vi "Create Plot Object.vi"(6 "Control Ref Queue":T1, 7 "Actual Transform In":T2, 8 "error in (no error)":errorcluster, 9 "Multiplot Representation In":T4, 10 "3D Stem.lvclass in":refnum<class "3D Scatter.lvclass">, 11 "Plot Object In":refnum<vi>) -> (0 "error out":errorcluster, 1 "Multiplot Representation Out":T4, 2 "3D Stem.lvclass out":refnum<class "3D Scatter.lvclass">, 3 "Plot Object Out":refnum<vi>, 5 "Actual Transform Out":T2)   [LabVIEW 2020, in "3D Scatter.lvclass"]
uses:
  <vilib>/Math Plots/3D Math Plots/3D Scatter/3D Scatter/3D Scatter.lvclass
  <vilib>/Math Plots/3D Math Plots/3D Plot/3D Plot/Typedef/Multiplot Representation.ctl
  <vilib>/Math Plots/3D Math Plots/3D Plot/3D Plot/Typedef/Plot Representation.ctl
  <vilib>/Math Plots/3D Math Plots/3D Plot/3D Plot/Typedef/Range Clusters.ctl
  <vilib>/Math Plots/3D Math Plots/3D Plot/3D Plot/Typedef/Mesh Data.ctl
  <vilib>/Math Plots/3D Math Plots/3D Plot/3D Plot/Typedef/Actual Transform.ctl
  <vilib>/Math Plots/3D Math Plots/3D Plot/Action String/3DMathPlot Ctrl Act Queue.ctl
  <vilib>/Math Plots/3D Math Plots/3D Plot/Action String/3DMathPlot Ctrl Act Cluster.ctl
  <vilib>/Math Plots/3D Math Plots/3D Plot/Action String/3DMathPlot State Class.ctl
  <vilib>/Math Plots/3D Math Plots/3D Scatter/3D Scatter/3D Scatter.lvclass/3D Scatter.ctl
  <vilib>/Math Plots/3D Math Plots/3D Plot/3D Plot/3D Plot.lvclass
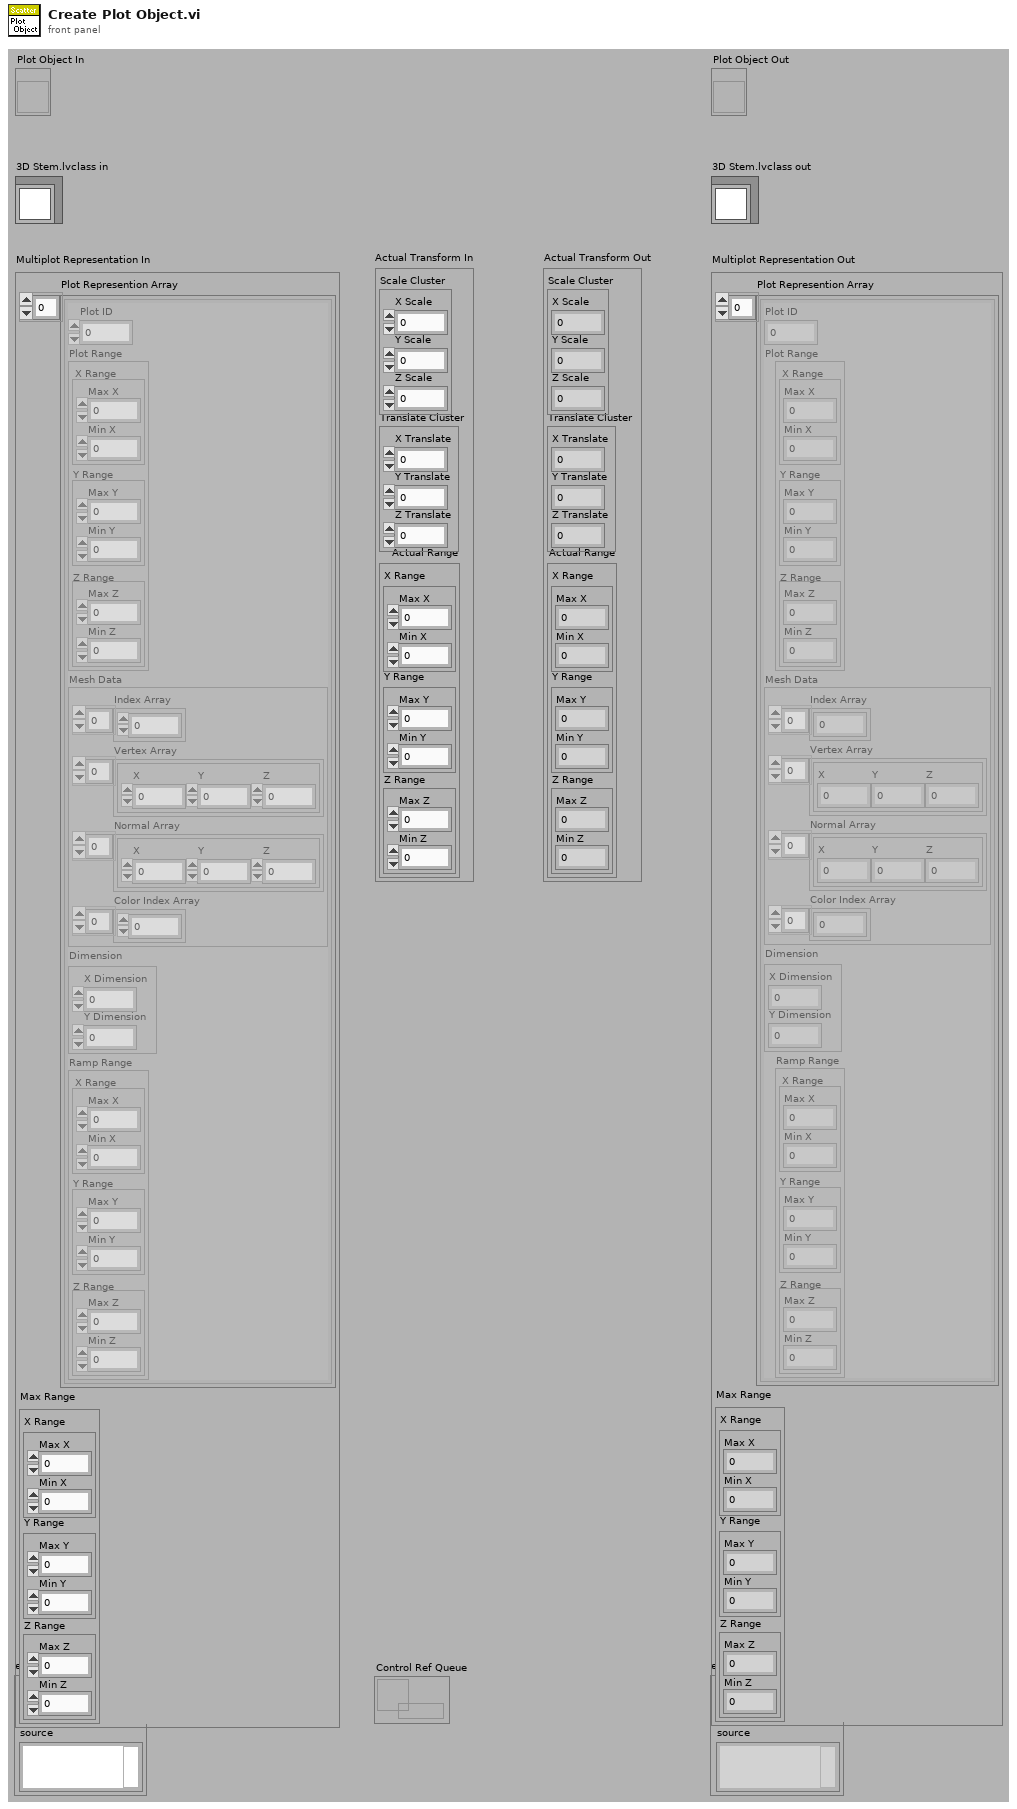
[diagram p1: front panel]
types:
  T1 = typedef "3DMathPlot Ctrl Act Queue.ctl" = refnum<queue>
  T2 = typedef "3D Plot.lvclass/Actual Transform.ctl" = cluster{"Scale Cluster":cluster{"X Scale":sgl, "Y Scale":sgl, "Z Scale":sgl}, "Translate Cluster":cluster{"X Translate":sgl, "Y Translate":sgl, "Z Translate":sgl}, "Actual Range":T3}
  T3 = typedef "3D Plot.lvclass/Range Clusters.ctl" = cluster{"X Range":cluster{"Max X":sgl, "Min X":sgl}, "Y Range":cluster{"Max Y":sgl, "Min Y":sgl}, "Z Range":cluster{"Max Z":sgl, "Min Z":sgl}}
  T4 = typedef "3D Plot.lvclass/Multiplot Representation.ctl" = cluster{"Plot Represention Array":T5[], "Max Range":T3}
  T5 = typedef "3D Plot.lvclass/Plot Representation.ctl" = cluster{"Plot ID":i32, "Plot Range":T3, "Mesh Data":T6, "Dimension":cluster{"X Dimension":i32, "Y Dimension":i32}, "Ramp Range":T3}
  T6 = typedef "3D Plot.lvclass/Mesh Data.ctl" = cluster{"Index Array":u32[], "Vertex Array":cluster{"X":sgl, "Y":sgl, "Z":sgl}[], "Normal Array":cluster{"X":sgl, "Y":sgl, "Z":sgl}[], "Color Index Array":i32[]}
  T7 = typedef "3D Scatter.lvclass/3D Scatter Property Array.ctl" = T8[]
  T8 = typedef "3D Scatter.lvclass/3D Scatter Property.ctl" = cluster{"General Property":cluster{"Plot Name":string, "Coordinate System":enum16{"Cartesian", "Cylindrical", "Spherical"}, "Opacity":sgl}, "Projection Property":cluster{"Draw XY":bool, "Draw YZ":bool, "Draw XZ":bool}, "Plot Property":cluster{"Sprite Type":T9, "Point Size":sgl, "Color Ramp Cluster":T10}}
  T9 = typedef "3D Plot.lvclass/Sprite Type.ctl" = enum16{"None", "Empty Square", "Solid Square", "Empty Diamond", "Solid Diamond", "Empty Circle", "Solid Circle", "Asterisk", "Bold X", "Wireframe Sphere", "Solid Sphere", "Wireframe Cube", "Solid Cube"}
  T10 = typedef "3D Plot.lvclass/Color Ramp Cluster.ctl" = cluster{"Color Ramp Style":enum16{"None", "Shaded", "Color spectrum", "Grey scale", "Custom"}, "Color Ramp Array":u32[], "Color Ramp Index":i32[], "Interpolate?":bool, "Logarithm?":bool}
  T11 = cluster{"Draw XY":bool, "Draw YZ":bool, "Draw XZ":bool}
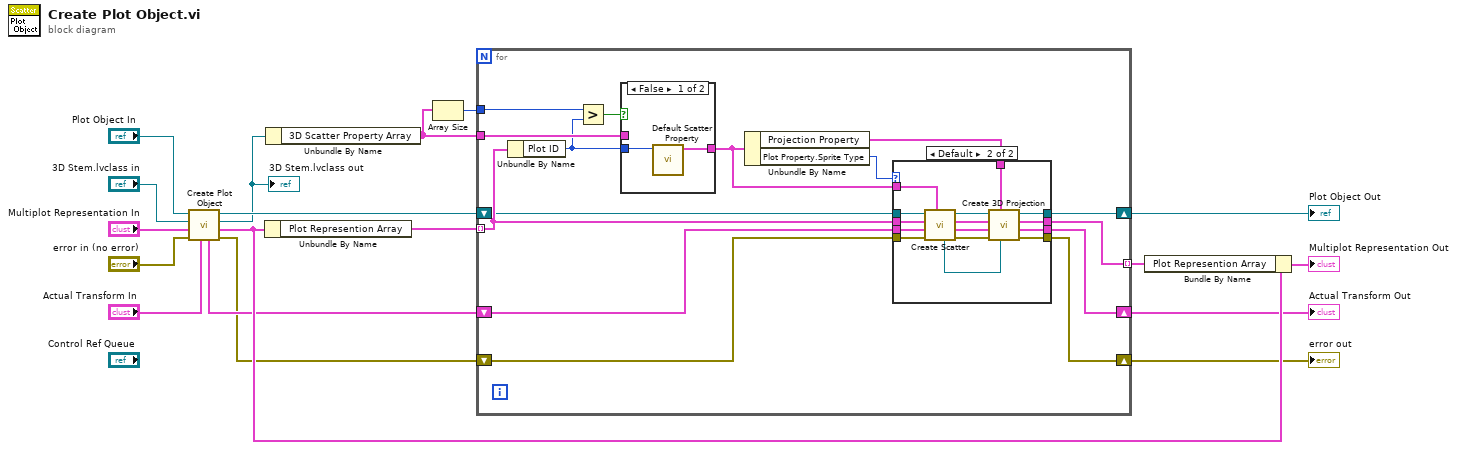
[diagram p0: block diagram]
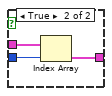
[diagram p2: hidden frame]
diagram:
  n1 = call-parent "Create Plot Object.vi"("Actual Transform In"="Actual Transform In", "error in (no error)"="error in (no error)", "Multiplot Representation In"="Multiplot Representation In", "3D Plot.lvclass in"="3D Stem.lvclass in", "Plot Object In"="Plot Object In") -> ("error out"=w3:errorcluster, "Multiplot Representation Out"=w12:T4, "3D Plot.lvclass out"=w4:refnum<class "3D Scatter.lvclass">, "Plot Object Out"=w6:refnum<vi>, "Actual Transform Out"=w9:T2)  [unwired: 2 in]
  "3D Stem.lvclass out" <- w4
  n2 = Unbundle By Name(w12) -> ("Plot Represention Array"=w14:T5[])
  n3 = Unbundle By Name(w4) -> ("3D Scatter Property Array"=w2:T7)
  n4 = Array Size(array=w2) -> (size(s)=w1:i32)
  n5 = for {
    shift-right: [w31] -> w7
    shift-left: w3 -> [w26]
    shift-right: [w33] -> w5
    shift-left: w6 -> [w28]
    shift-right: [w32] -> w8
    shift-left: w9 -> [w27]
    tunnel: w14 -> [w29] mode=indexing
    tunnel: w2 -> [w22]
    tunnel: [w30] -> w13 mode=indexing
    tunnel: w1 -> [w19]
    n6 = Unbundle By Name(w29) -> ("Plot ID"=w21:i32)
    n7 = Greater?(x=w19, y=w21) -> (0:w23:bool)
    n8 = case shown="False" w23 {
      tunnel: w22 -> [_ w38]
      tunnel: [w34 w37] -> w20
      tunnel: w21 -> [w35 w36]
      frame False {
        n9 = call <vilib>:"Default Scatter Property.vi"("Plot ID"=w35) -> ("Default Property"=w34:T8)  [unwired: 10 out]
      }
      frame True {
        n10 = Index Array(array=w38, index=w36) -> (element=w37:T8)
      }
    }
    n11 = Unbundle By Name(w20) -> ("Projection Property"=w25:T11, "Plot Property.Sprite Type"=w24:T9)
    n12 = case shown="Default" w24 {
      tunnel: [w42 w56] -> w33
      tunnel: [w40 w55] -> w32
      tunnel: [w39 w54] -> w31
      tunnel: [w41 w51] -> w30
      tunnel: w29 -> [w41 w48]
      tunnel: w28 -> [w42 w47]
      tunnel: w27 -> [w40 w46]
      tunnel: w26 -> [w39 w45]
      tunnel: w25 -> [_ w44]
      tunnel: w20 -> [_ w43]
      frame "None" {
      }
      frame Default {
        n13 = call <vilib>:"Create Scatter.vi"("3D Scatter Property"=w43, "error in (no error)"=w45, "Actual Transform In"=w46, "Plot Representation In"=w48, "Plot Object In"=w47) -> ("error out"=w53:errorcluster, "Actual Transform Out"=w52:T2, "Plot Representation Out"=w51:T5, "Plot Object Out"=w50:refnum<vi>, "Scatter Object Out"=w49:refnum<vi>)  [unwired: 1 in, 1 out]
        n14 = call <vilib>:"Create 3D Projection.vi"("Sub Object In"=w49, "Projection Property"=w44, "error in (no error)"=w53, "Actual Transform In"=w52, "Plot Object In"=w50) -> ("error out"=w54:errorcluster, "Actual Transform Out"=w55:T2, "Plot Object Out"=w56:refnum<vi>)  [unwired: 1 in, 3 out]
      }
    }
  }
  "error out" <- w7
  "Plot Object Out" <- w5
  "Actual Transform Out" <- w8
  n15 = Bundle By Name(cluster=w12, "Plot Represention Array"=w13) -> (→"Multiplot Representation Out":T4)
